vi "ServiceChannels.Create.vi"(8 "error in (no error)":errorcluster, 11 "nodeID in":T1 format="%.0x") -> (0 "error out":errorcluster, 3 "nodeID out":u64)   [LabVIEW 2024, in "Diagnostics Addon System Explorer.lvlib"]
uses:
  Diagnostics Addon System Explorer.lvlib
  <vilib>/NI VeriStand/Custom Device API/Custom Device Item Ref.ctl
  <vilib>/NI VeriStand/Custom Device API/Custom Device Channel.ctl
  <vilib>/NI VeriStand/Custom Device API/Custom Device Channel Type.ctl
  Addon Shared/SubVIs/Constants.vi
  <vilib>/NI/NI VeriStand Advanced SysDef API/SysDef API/Advanced System Definition.lvlib
  Addon Shared/Diagnostics Addon Shared.lvlib
  <vilib>/NI VeriStand/Custom Device API/Custom Device API.lvlib
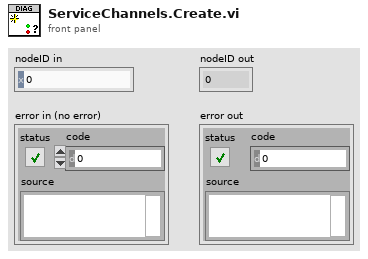
[diagram p1: front panel]
types:
  T1 = typedef "Custom Device API.lvlib/Custom Device Item Ref.ctl" = u64
  T2 = typedef "Custom Device API.lvlib/Custom Device Channel.ctl" = cluster{"Type":T3, "Units":string, "Default Value":dbl, "Faultable":bool, "Scalable":bool}
  T3 = typedef "Custom Device API.lvlib/Custom Device Channel Type.ctl" = enum16{"Input", "Output"}
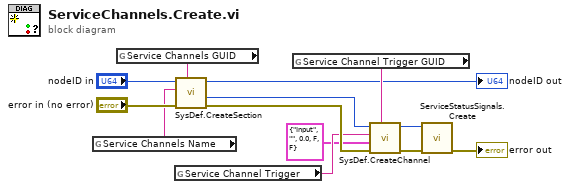
[diagram p0: block diagram]
diagram:
  n1 = global read "Constants.vi" "Service Channels Name"() -> (w4:string)
  n2 = global read "Constants.vi" "Service Channels GUID"() -> (w8:string)
  n3 = global read "Constants.vi" "Service Channel Trigger"() -> (w10:string)
  n4 = call <vilib>:"SysDef.CreateSection.vi"("GUID"=w8, "error in (no error)"="error in (no error)", "Name"=w4, "nodeID"="nodeID in") -> ("error out"=w12:errorcluster, "New NodeID"=w13:u64, "nodeID out"=→"nodeID out":u64)  [unwired: 4 in, 1 out]
  n5 = global read "Constants.vi" "Service Channel Trigger GUID"() -> (w11:string)
  n6 = call <vilib>:"SysDef.CreateChannel.vi"("GUID"=w11, "error in (no error)"=w12, "Channel"=T2 {"Type"=enum."Input", "Units"="", "Default Value"=0.0, "Faultable"=FALSE, "Scalable"=FALSE}, "Name"=w10, "nodeID"=w13) -> ("error out"=w3:errorcluster, "nodeID out"=w2:u64)  [unwired: 3 in, 2 out]
  n7 = call "ServiceStatusSignals.Create.vi"("error in (no error)"=w3, "nodeID in"=w2) -> ("error out"=→"error out":errorcluster)  [unwired: 8 in, 1 out]
